vi "InjectChild.vi"(8 "error in (no error)":errorcluster, 10 "Child":refnum<class "Class.lvclass">, 11 "Interface in":refnum<class "Interface.lvclass">) -> (0 "error out":errorcluster, 3 "Interface out":refnum<class "Interface.lvclass">)   [LabVIEW 2020, in "Mermaid.lvlib" / "Interface.lvclass"]
uses:
  Interface.lvclass
  _Class/Class.lvclass
  Interface.lvclass/Interface.ctl
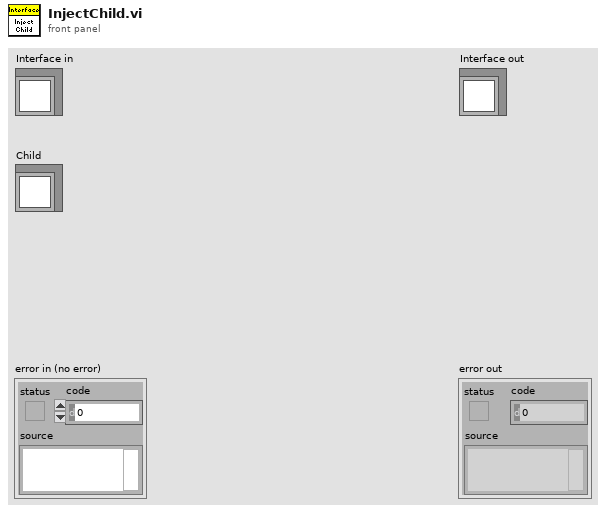
[diagram p1: front panel]
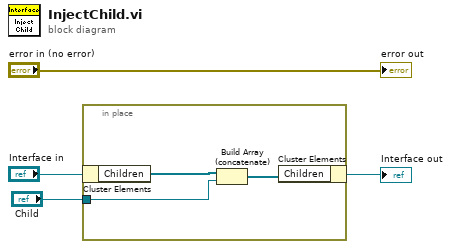
[diagram p0: block diagram]
diagram:
  n1 = in-place {
    in-place-border: "Child" -> [w6]
    n2 = in-place-cluster #1("Interface in") -> ("Children"=w7:refnum<class "Class.lvclass">[])
    n3 = Build Array (concatenate)(w7, w6) -> (w5:refnum<class "Class.lvclass">[])
    n4 = in-place-cluster #1("Children"=w5) -> (→"Interface out":refnum<class "Interface.lvclass">)
  }
  "error out" <- "error in (no error)"
